vi "XW quadrant analysis, PN.vi"(0 "V":dbl[](array[numeric]), 1 "Umean":dbl, 2 "Vmean":dbl, 3 "No. of blocks":i32, 4 "U":dbl[](array[numeric])) -> (5 "Quadrant probability":dbl[](array[numeric]))   [LabVIEW 2010]
panel:
  # "Q 0, 0 : uv --"
  # "Q 0, 1 : uv -+"
  # "Q 1, 0 : uv +-"
  # "Q 1, 1 : uv ++"
  # "N.B. The values of Umean and Vmean MUST be those of the ENTIRE dataset (i.e. all blocks) otherwise this routine will be inconsistent and therefore tell lies to you!!\n\nTo use this vi in a block by block manner, take note of the above and then simply add the resulting array from each block as you go."
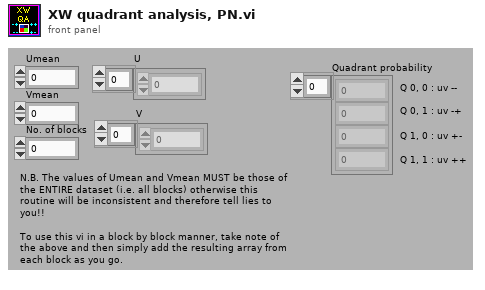
[diagram p1: front panel]
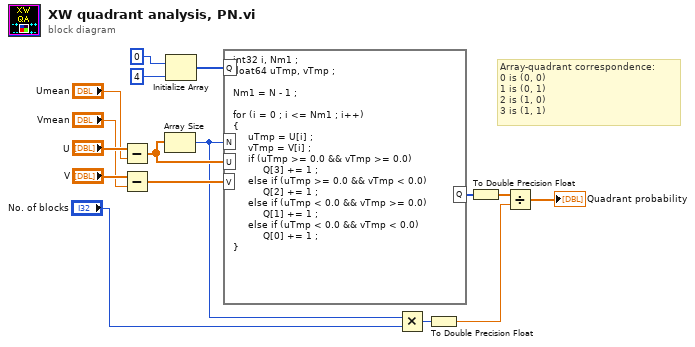
[diagram p0: block diagram]
diagram:
  # "Array-quadrant correspondence:\n0 is (0, 0)\n1 is (0, 1)\n2 is (1, 0)\n3 is (1, 1)"
  n1 = Subtract(x="U", y="Umean") -> (x-y=w9:dbl[])
  n2 = Subtract(x="V", y="Vmean") -> (x-y=w10:dbl[])
  n3 = Array Size(array=w9) -> (size(s)=w6:i32)
  n4 = Initialize Array(0 ("element"), 4 ("dimension size")) -> (w11:i32[])
  n5 = formula code="int32 i, Nm1 ;\nfloat64 uTmp, vTmp ;\n\nNm1 = N - 1 ;\n\nfor (i = 0 ; i <= Nm1 ; i++)\n{\n     uTmp = U[i] ;\n     vTmp = V[i] ;\n     if (uTmp >= 0.0 && vTmp >= 0.0)\n          Q[3] += 1 ;\n     else if (uTmp >= 0.0 && vTmp < 0.0)\n          Q[2] += 1 ;\n     else if (uTmp < 0.0 && vTmp >= 0.0)\n          Q[1] += 1 ;\n     else if (uTmp < 0.0 && vTmp < 0.0)\n          Q[0] += 1 ;\n}"("N"=w6, "Q"=w11, "U"=w9, "V"=w10) -> ("Q"=w5:i32[])
  n6 = Multiply(x=w6, y="No. of blocks") -> (x*y=w4:i32)
  n7 = To Double Precision Float(number=w4) -> (double precision float=w3:dbl)
  n8 = To Double Precision Float(number=w5) -> (double precision float=w2:dbl[])
  n9 = Divide(x=w2, y=w3) -> (x/y=→"Quadrant probability":dbl[])
